vi "Init.vi"(8 "error in (no error)":errorcluster, 11 "AI_Snake in":refnum<class "AI_Snake.lvclass">) -> (0 "error out":errorcluster, 3 "AI_Snake out":refnum<class "AI_Snake.lvclass">)   [LabVIEW 2019, in "RT_Game.lvlib" / "AI_Snake.lvclass"]
uses:
  AI_Snake.lvclass
  Snake/Snake.lvclass
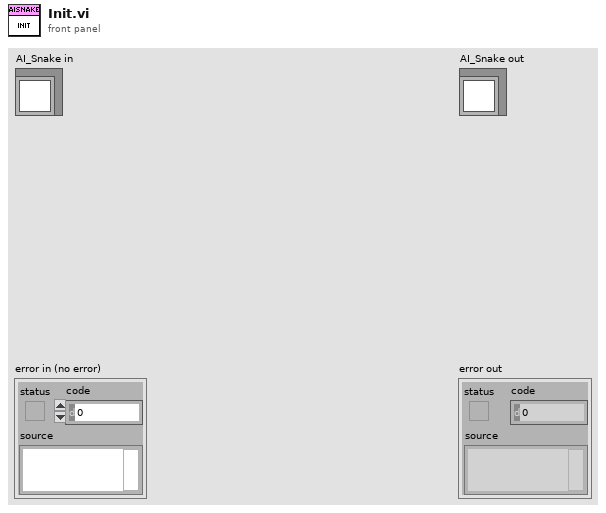
[diagram p1: front panel]
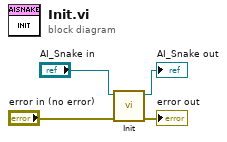
[diagram p0: block diagram]
diagram:
  n1 = call-parent "Init.vi"("error in (no error)"="error in (no error)", "Snake in"="AI_Snake in") -> ("error out"=→"error out":errorcluster, "Snake out"=→"AI_Snake out":refnum<class "AI_Snake.lvclass">)  [unwired: 8 in]
